vi "calc polar to rect.vi"(7 "units":enum16{"degrees", "radians"}(ring), 10 "angle":dbl, 11 "mag":dbl) -> (3 "XY":cluster{"X":dbl, "Y":dbl})   [LabVIEW 2023]
panel:
  out "X":dbl
  out "Y":dbl
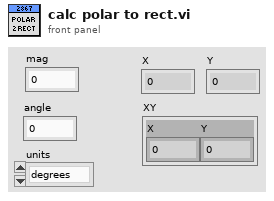
[diagram p1: front panel]
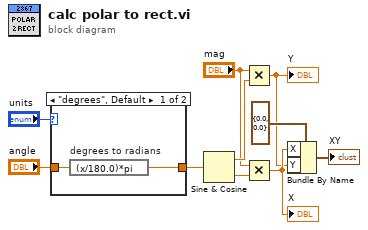
[diagram p0: block diagram]
diagram:
  n1 = case shown="\"degrees\", Default" "units" {
    tunnel: "angle" -> [w12 w13]
    tunnel: [w11 w13] -> w3
    frame "degrees", Default {
      n2 = expression code="(x/180.0)*pi" "degrees to radians"(w12) -> (w11:dbl)
    }
    frame "radians" {
    }
  }
  n3 = Sine & Cosine(0:w3) -> (1:w10:dbl, 2:w9:dbl)
  n4 = Multiply(x="mag", y=w10) -> (x*y=w4:dbl)
  "Y" <- w4
  n5 = Multiply(x="mag", y=w9) -> (x*y=w5:dbl)
  "X" <- w5
  n6 = Bundle By Name(cluster=cluster{"X":dbl, "Y":dbl} {"X"=0.0, "Y"=0.0} ("XY"), "X"=w5, "Y"=w4) -> (→"XY":cluster{"X":dbl, "Y":dbl})
